vi "Base Run Tool.vi"(4 "cmdline in error in":bool, 5 "use tools path in":bool, 6 "working directory in":string, 7 "error in":errorcluster, 8 "tool args in":string, 9 "tool path in":string, 10 "ATS Framework Fields in":T2) -> (0 "error out":errorcluster, 2 "run tool output":T1, 3 "ATS Framework Fields out":T2)   [LabVIEW 2022 SP3]
uses:
  ATS Framework Fields.ctl
  Run Tool Output.ctl
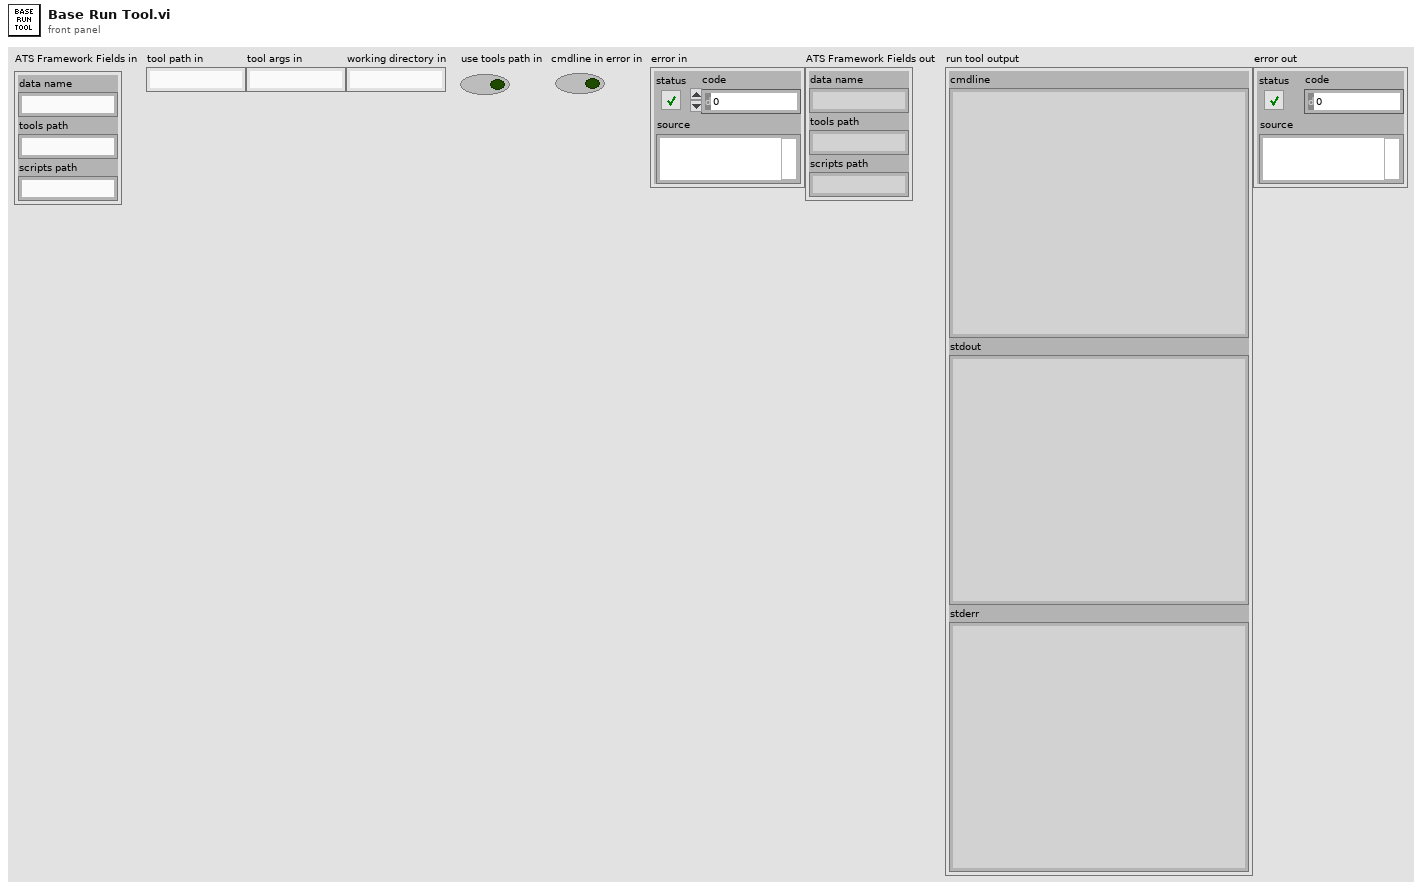
[diagram p1: front panel]
types:
  T1 = typedef "Run Tool Output.ctl" = cluster{"cmdline":string, "stdout":string, "stderr":string}
  T2 = typedef "ATS Framework Fields.ctl" = cluster{"data name":string, "tools path":string, "scripts path":string}
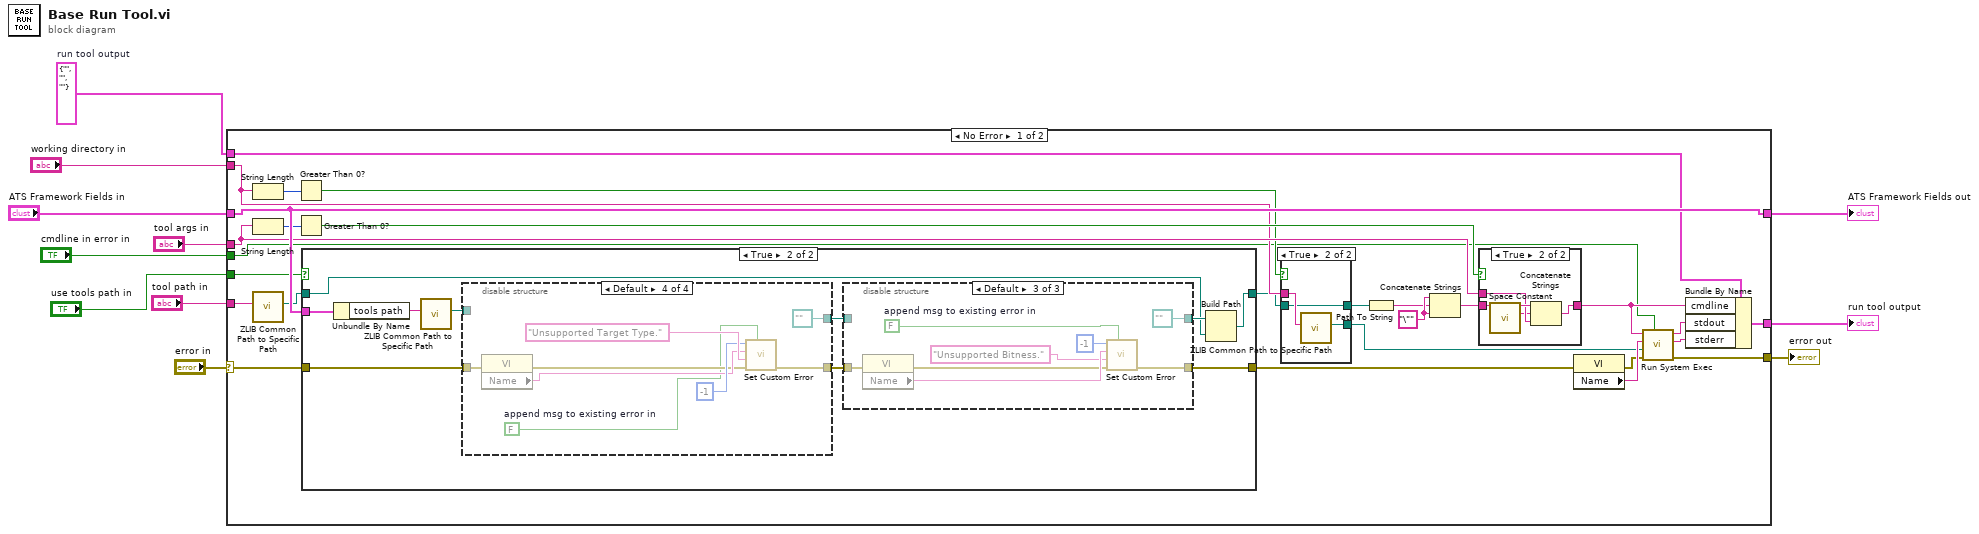
[diagram p0: block diagram]
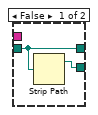
[diagram p2: hidden frame]
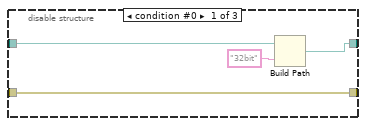
[diagram p4: hidden frame]
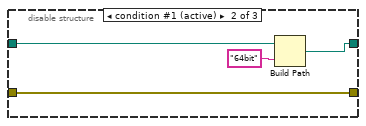
[diagram p5: hidden frame]
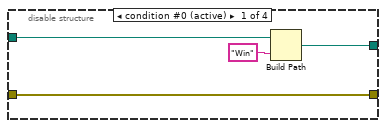
[diagram p6: hidden frame]
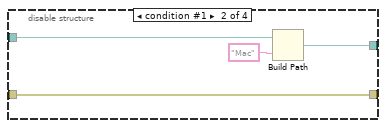
[diagram p7: hidden frame]
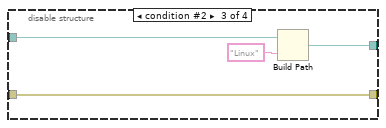
[diagram p8: hidden frame]
diagram:
  w5 = T1 {"cmdline"="", "stdout"="", "stderr"=""}  # run tool output
  n1 = case shown="No Error" "error in" {
    selector: "error in" -> [w37 w99]
    tunnel: [w23 w99] -> w11
    tunnel: "tool args in" -> [w30 _]
    tunnel: "ATS Framework Fields in" -> [w36 w98]
    tunnel: "tool path in" -> [w21 _]
    tunnel: [w36 w98] -> w6
    tunnel: [w35 w97] -> w4
    tunnel: w5 -> [w34 w97]
    tunnel: "use tools path in" -> [w22 _]
    tunnel: "working directory in" -> [w18 _]
    tunnel: "cmdline in error in" -> [w12 _]
    frame No Error {
      w38 = "\"" ("string")
      n2 = String Length(string=w18) -> (length=w17:i32)
      n3 = String Length(string=w30) -> (length=w33:i32)
      n4 = call "ZLIB Common Path to Specific Path.vi"("common path"=w21) -> ("specific path"=w20:path)  [unwired: 10 in]
      n5 = Greater Than 0?(x=w17) -> (x > 0?=w16:bool)
      n6 = Greater Than 0?(x=w33) -> (x > 0?=w32:bool)
      n7 = case shown="True" w22 {
        tunnel: [w44 w46] -> w14
        tunnel: w37 -> [w45 w54]
        tunnel: w36 -> [_ w50]
        tunnel: [w45 w49] -> w27
        tunnel: w20 -> [w44 w47]
        frame False {
        }
        frame True {
          n8 = Unbundle By Name(w50) -> ("tools path"=w55:string)
          n9 = call "ZLIB Common Path to Specific Path.vi"("common path"=w55) -> ("specific path"=w48:path)  [unwired: 10 in]
          n10 = disable-structure shown="Default" {
            disable-tunnel: w54 -> [w75 w79 w83 w86]
            disable-tunnel: [w75 w79 w83 w90] -> w52
            disable-tunnel: w48 -> [w74 w78 w82 _]
            disable-tunnel: [w73 w77 w81 path "" ("appended path")] -> w53
            frame condition #0 (active) {
              n11 = Build Path(base path=w74, name or relative path="Win") -> (appended path=w73:path)
            }
            frame condition #1 {
              n12 = Build Path(base path=w78, name or relative path="Mac") -> (appended path=w77:path)
            }
            frame condition #2 {
              n13 = Build Path(base path=w82, name or relative path="Linux") -> (appended path=w81:path)
            }
            frame condition #3 {
              w84 = FALSE  # append msg to existing error in
              n14 = property class="VI"(error in=w86) -> (error out=w85:errorcluster, "Name"=w87:string)  [unwired: 1 in, 1 out]
              n15 = call "Set Custom Error.vi"("append msg to existing error in"=w84, "error in"=w85, "message in"="Unsupported Target Type." ("source"), "source in"=w87, "code in"=-1 ("code")) -> ("error out"=w90:errorcluster)  [unwired: 6 in]
            }
          }
          n16 = disable-structure shown="Default" {
            disable-tunnel: w52 -> [w59 w62 w66]
            disable-tunnel: [w59 w62 w65] -> w49
            disable-tunnel: w53 -> [w58 w61 _]
            disable-tunnel: [w57 w60 path "" ("appended path")] -> w51
            frame condition #0 {
              n17 = Build Path(base path=w58, name or relative path="32bit") -> (appended path=w57:path)
            }
            frame condition #1 (active) {
              n18 = Build Path(base path=w61, name or relative path="64bit") -> (appended path=w60:path)
            }
            frame condition #2 {
              w64 = FALSE  # append msg to existing error in
              n19 = property class="VI"(error in=w66) -> (error out=w68:errorcluster, "Name"=w69:string)  [unwired: 1 in, 1 out]
              n20 = call "Set Custom Error.vi"("append msg to existing error in"=w64, "error in"=w68, "message in"="Unsupported Bitness." ("source"), "source in"=w69, "code in"=-1 ("code")) -> ("error out"=w65:errorcluster)  [unwired: 6 in]
            }
          }
          n21 = Build Path(base path=w51, name or relative path=w47) -> (appended path=w46:path)
        }
      }
      n22 = case shown="True" w16 {
        tunnel: w18 -> [_ w43]
        tunnel: [w40 w42] -> w15
        tunnel: w14 -> [w39 w41]
        tunnel: [w39 w41] -> w13
        frame False {
          n23 = Strip Path(path=w39) -> (stripped path=w40:path)  [unwired: 1 out]
        }
        frame True {
          n24 = call "ZLIB Common Path to Specific Path.vi"("common path"=w43) -> ("specific path"=w42:path)  [unwired: 10 in]
        }
      }
      n25 = Path To String(path=w13) -> (string=w19:string)
      n26 = Concatenate Strings(w38, w19, w38) -> (w31:string)
      n27 = case shown="True" w32 {
        tunnel: w31 -> [w92 w96]
        tunnel: [w92 w95] -> w29
        tunnel: w30 -> [_ w94]
        frame False {
        }
        frame True {
          n28 = call <vilib>:"Space Constant.vi"() -> ("String"=w93:string)
          n29 = Concatenate Strings(w96, w93, w94) -> (w95:string)
        }
      }
      n30 = property class="VI"(error in=w27) -> (error out=w26:errorcluster, "Name"=w28:string)  [unwired: 1 in, 1 out]
      n31 = call "Run System Exec.vi"("cmdline in error in"=w12, "error in"=w26, "working directory in"=w15, "vi name in"=w28, "command in"=w29) -> ("error out"=w23:errorcluster, "standard error out"=w24:string, "standard output out"=w25:string)  [unwired: 4 in]
      n32 = Bundle By Name(cluster=w34, "cmdline"=w29, "stdout"=w25, "stderr"=w24) -> (w35:T1)
    }
    frame Error {
    }
  }
  "error out" <- w11
  "ATS Framework Fields out" <- w6
  "run tool output" <- w4
